vi "LvMPDC_SUB_PlaybackOptionPanel.vi"(10 "Playback option":T1) -> (1 "Cancel?":bool, 2 "Playback option out":T1)   [LabVIEW 2012]
uses:
  LvMPDC_Typdef_PlaybackOption.ctl
  <vilib>/Utility/miscctls.llb/LVPointTypeDef.ctl
panel:
  in  "chk repeat":bool
  in  "btn Cancel":bool
  in  "btn OK":bool
  in  "chk single":bool
  in  "chk random":bool
  in  "chk consume":bool
  in  "chk crossfade":bool
  # "Playback Option"
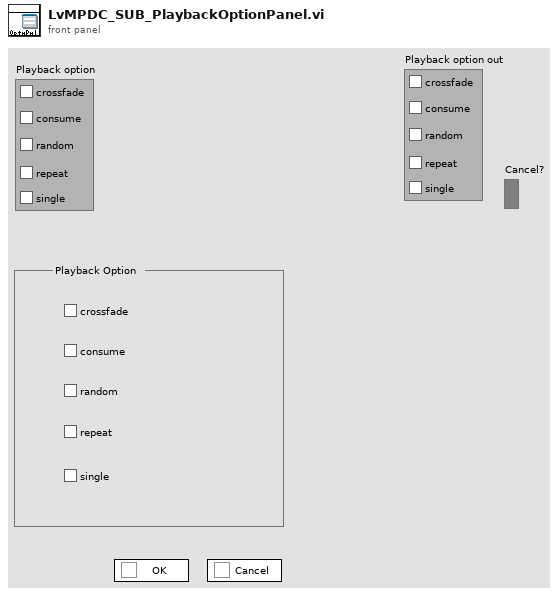
[diagram p1: front panel]
types:
  T1 = typedef "LvMPDC_Typdef_PlaybackOption.ctl" = cluster{"chk crossfade":bool, "chk consume":bool, "chk random":bool, "chk repeat":bool, "chk single":bool}
  T2 = typedef "LVPointTypeDef.ctl" = cluster{"Horizontal":i16, "Vertical":i16}
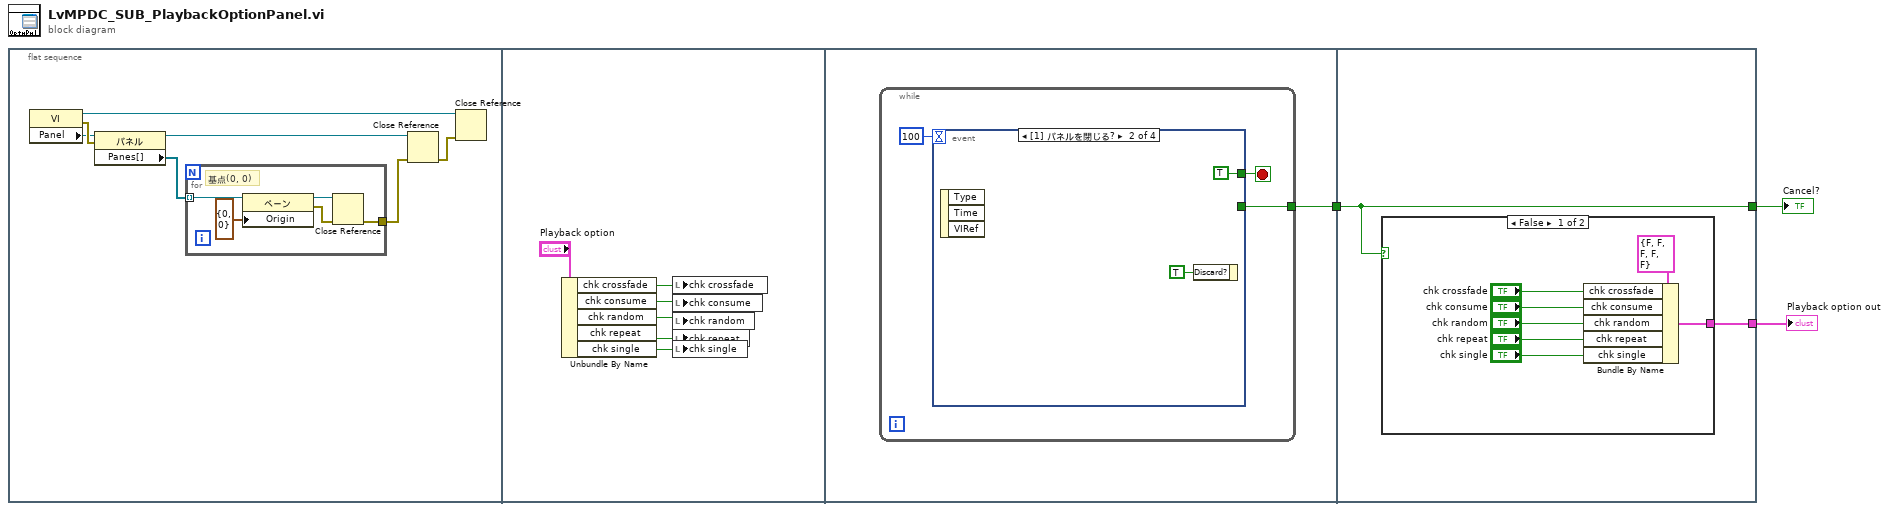
[diagram p0: block diagram]
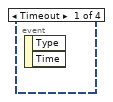
[diagram p2: hidden frame]
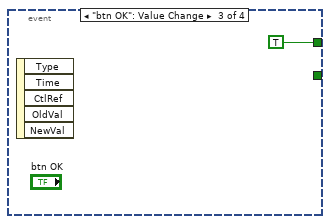
[diagram p3: hidden frame]
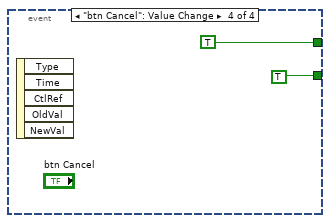
[diagram p4: hidden frame]
diagram:
  n1 = flat-sequence {
    tunnel: [w22] -> w3
    tunnel: [w32] -> w2
    tunnel: w3 -> [w32]
    tunnel: [w31] -> w1
    frame #0 {
      n2 = property class="VI"() -> (reference out=w7:refnum<vi>, error out=w10:errorcluster, "Panel"=w4:refnum<vi>)  [unwired: 2 in]
      n3 = property on="プロパティノード" class="パネル"(reference=w4, error in=w10) -> (reference out=w6:refnum<vi>, "Panes[]"=w5:refnum<vi>[])  [unwired: 1 out]
      n4 = for {
        tunnel: w5 -> [w15] mode=indexing
        tunnel: [w12] -> w8
        # "基点(0, 0)"
        n5 = property on="プロパティノード" class="ペーン"(reference=w15, "Origin"=T2 {"Horizontal"=0, "Vertical"=0} ("原点")) -> (reference out=w14:refnum<vi>, error out=w13:errorcluster)  [unwired: 1 in]
        n6 = Close Reference(reference=w14, error in (no error)=w13) -> (error out=w12:errorcluster)
      }
      n7 = Close Reference(reference=w6, error in (no error)=w8) -> (error out=w9:errorcluster)
      n8 = Close Reference(reference=w7, error in (no error)=w9) -> ()  [unwired: 1 out]
    }
    frame #1 {
      n9 = Unbundle By Name("Playback option") -> ("chk crossfade"=w20:bool, "chk consume"=w19:bool, "chk random"=w18:bool, "chk repeat"=w16:bool, "chk single"=w17:bool)
      n10 = local write "chk crossfade"(w20) -> ()
      n11 = local write "chk consume"(w19) -> ()
      n12 = local write "chk random"(w18) -> ()
      n13 = local write "chk repeat"(w16) -> ()
      n14 = local write "chk single"(w17) -> ()
    }
    frame #2 {
      n15 = while {
        tunnel: [w23] -> w22
        stop <- w24 stop-if-true
        n16 = event shown="[1] パネルを閉じる?" {
          selector: _ -> [_ _ _ _]
          dyn-events: _ -> [_ _ _ _]
          timeout: 100 -> [_ _ _ _]
          tunnel: [_ TRUE TRUE TRUE] -> w24
          tunnel: [_ _ _ TRUE] -> w23
          event Timeout {
            n17 = event-data() -> ()  [unwired: 1 in, 2 out]
          }
          event Panel Close? {
            n18 = event-data() -> ()  [unwired: 1 in, 3 out]
            n19 = event-data("Discard?"=TRUE ("破棄?")) -> ()  [unwired: 1 in, 1 out]
          }
          event "btn OK": Value Change {
            n20 = event-data() -> ()  [unwired: 1 in, 5 out]
          }
          event "btn Cancel": Value Change {
            n21 = event-data() -> ()  [unwired: 1 in, 5 out]
          }
        }
      }
    }
    frame #3 {
      n22 = case shown="FALSE" w32 {
        tunnel: [w34 _] -> w31
        frame False {
          n23 = Bundle By Name(cluster=T1 {"chk crossfade"=FALSE, "chk consume"=FALSE, "chk random"=FALSE, "chk repeat"=FALSE, "chk single"=FALSE} ("Playback option out"), "chk crossfade"="chk crossfade", "chk consume"="chk consume", "chk random"="chk random", "chk repeat"="chk repeat", "chk single"="chk single") -> (w34:T1)
        }
        frame True {
        }
      }
    }
  }
  "Playback option out" <- w1
  "Cancel?" <- w2
